vi "zmq_socket_check.vi"(1 "socket in":refnum<class "Socket.lvclass">) -> (0 "valid?":bool)   [LabVIEW 2025, in "ZeroMQ.lvlib" / "Socket.lvclass"]
doc: "Checks whether the supplied socket object is valid"
uses:
  Socket.lvclass
  Socket.lvclass/Socket.ctl
  ZeroMQ.lvlib
panel:
  # "ØMQ"
  # "labview"
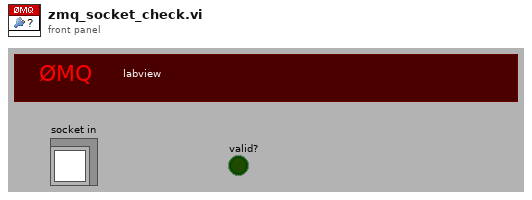
[diagram p1: front panel]
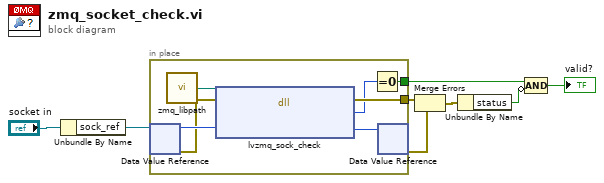
[diagram p0: block diagram]
diagram:
  n1 = Unbundle By Name("socket in") -> ("sock_ref"=w1:refnum<data-value>)
  n2 = in-place {
    in-place-border: [w11] -> w8
    in-place-border: [w9] -> w5
    n3 = in-place-dvr #1(w1) -> (w15:u64, w12:errorcluster)
    n4 = call "zmq_libpath.vi"() -> ("path"=w13:path)
    n5 = dll-call lib="?" fn="lvzmq_sock_check" ("zmq_labview.dll:lvzmq_socket")(path in=w13, error in=w12, "sock_obj"=w15) -> (error out=w11:errorcluster, "return type"=w10:i32, "sock_obj"=w14:u64)  [unwired: 1 in, 1 out]
    n6 = Equal To 0?(x=w10) -> (x = 0?=w9:bool)
    n7 = in-place-dvr #1(w14) -> (w7:errorcluster)  [unwired: 1 out]
  }
  n8 = Merge Errors(w8, w7) -> (w6:errorcluster)
  n9 = Unbundle By Name(w6) -> ("status"=w4:bool)
  n10 = Compound Arithmetic op=AND(w5, invert w4) -> (→"valid?":bool)
